vi "convert '' to NULL.vi"(0 "String In":string, 1 "length":i32=1000) -> (2 "Formatted String":string)   [LabVIEW 2020, in "hse-db-ado.lvlib" / "ADO-DB-Driver.lvlib"]
doc: "Convert an empty string (two quotes) to NULL\n\n____\nHAMPEL SOFTWARE ENGINEERING v1.4.0 (2023-12-19 09:52)"
uses:
  ADO-DB-Driver.lvlib
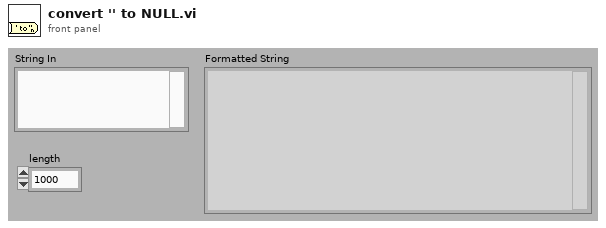
[diagram p1: front panel]
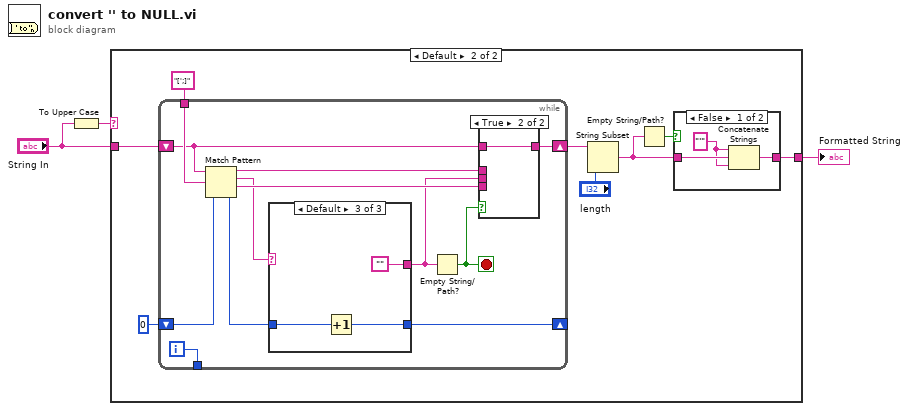
[diagram p0: block diagram]
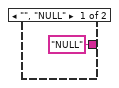
[diagram p2: hidden frame]
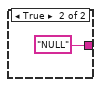
[diagram p3: hidden frame]
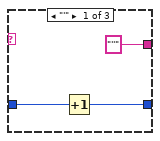
[diagram p4: hidden frame]
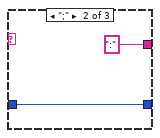
[diagram p5: hidden frame]
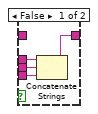
[diagram p6: hidden frame]
diagram:
  n1 = To Upper Case(1:"String In") -> (0:w1:string)
  n2 = case shown="Default" w1 {
    tunnel: "String In" -> [_ w12]
    tunnel: ["NULL" w7] -> w3
    frame "", "NULL" {
    }
    frame Default {
      n3 = while {
        tunnel: [w22] -> _
        shift-left: 0 ("offset past match") -> [w23]
        shift-right: [w19] -> _
        tunnel: "[';]" ("regular expression") -> [w25]
        shift-left: w12 -> [w24]
        shift-right: [w26] -> w9
        i -> [w22]
        stop <- w17 stop-if-true
        n4 = Match Pattern(string=w24, regular expression=w25, offset (0)=w23) -> (before substring=w27:string, match substring=w21:string, after substring=w28:string, offset past match=w20:i32)
        n5 = case shown="Default" w21 {
          tunnel: ["''" ("substitute string") ":" ("substitute string") ""] -> w18
          tunnel: w20 -> [w30 w32 w36]
          tunnel: [w29 w32 w35] -> w19
          frame "'" {
            n6 = Increment(x=w30) -> (x+1=w29:i32)
          }
          frame ";" {
          }
          frame Default {
            n7 = Increment(x=w36) -> (x+1=w35:i32)
          }
        }
        n8 = Empty String/Path?(string/path=w18) -> (empty?=w17:bool)
        n9 = case shown="True" w17 {
          tunnel: w18 -> [w40 _]
          tunnel: [w39 w41] -> w26
          tunnel: w27 -> [w38 _]
          tunnel: w28 -> [w37 _]
          tunnel: w24 -> [_ w41]
          frame False {
            n10 = Concatenate Strings(w38, w40, w37) -> (w39:string)
          }
          frame True {
          }
        }
      }
      n11 = String Subset(string=w9, length (rest)="length") -> (substring=w5:string)  [unwired: 1 in]
      n12 = Empty String/Path?(string/path=w5) -> (empty?=w6:bool)
      n13 = case shown="False" w6 {
        tunnel: w5 -> [w15 _]
        tunnel: [w14 "NULL"] -> w7
        frame False {
          w13 = "'" ("string")
          n14 = Concatenate Strings(w13, w15, w13) -> (w14:string)
        }
        frame True {
        }
      }
    }
  }
  "Formatted String" <- w3
